vi "front_panel_ctl_save.vi"(0 "VI in":refnum<vi>, 1 "method":enum16{"read controls", "write controls"}(ring), 2 "filename":path, 3 "controls":string[](array[string]), 5 "error in (no error)":errorcluster) -> (8 "error out":errorcluster)   [LabVIEW 2015]
uses:
  <vilib>/Utility/config.llb/Read Key (String).vi
  <vilib>/Utility/config.llb/Write Key (String).vi
  <vilib>/Utility/config.llb/NI_LVConfig.lvlib
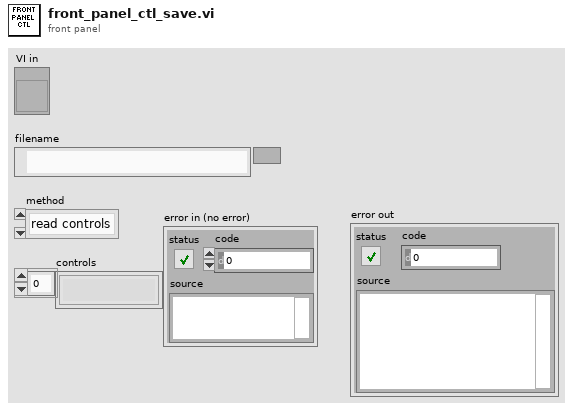
[diagram p1: front panel]
types:
  T1 = typedef "NI_LVConfig.lvlib/Config Data RefNum.ctl" = refnum<k1>
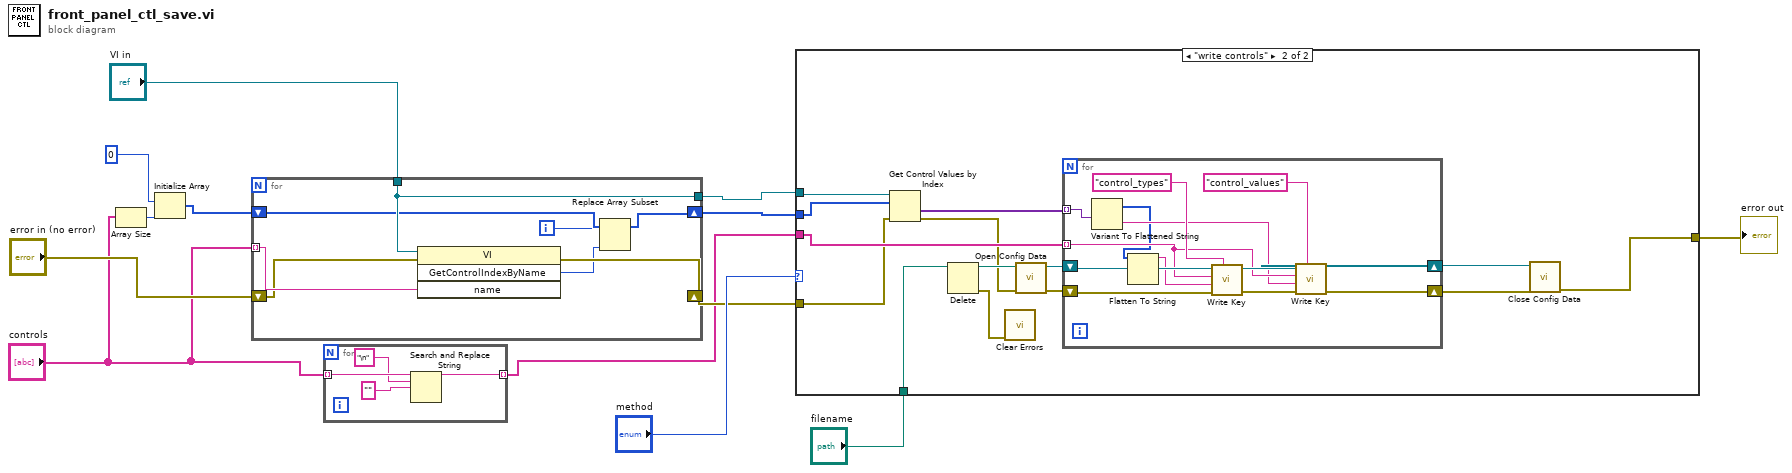
[diagram p0: block diagram]
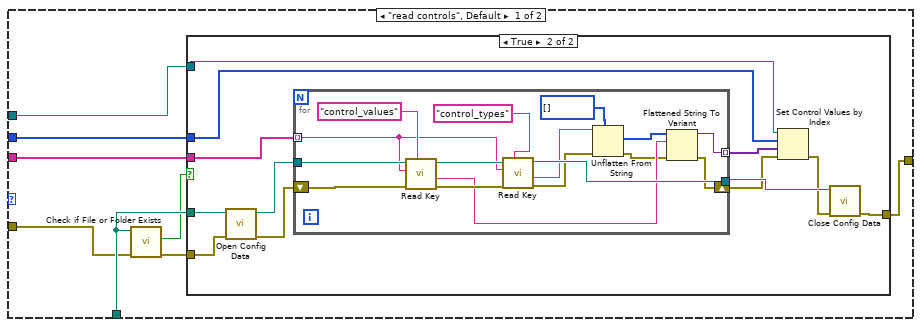
[diagram p2: hidden frame]
diagram:
  n1 = Array Size(array="controls") -> (size(s)=w4:i32)
  n2 = Initialize Array(0 ("Get Control Index by Name"), w4) -> (w2:i32[])
  n3 = for {
    tunnel: "controls" -> [w21] mode=indexing
    shift-right: [w16] -> w12
    shift-left: w2 -> [w17]
    tunnel: [w20] -> w11
    tunnel: "VI in" -> [w20]
    shift-right: [w19] -> w8
    shift-left: "error in (no error)" -> [w18]
    i -> [w15]
    n4 = invoke class="VI" method="GetControlIndexByName"(reference=w20, error in=w18, "name"=w21) -> (error out=w19:errorcluster, "GetControlIndexByName"=w14:i32)  [unwired: 1 in, 2 out]
    n5 = Replace Array Subset(array=w17, new element=w14, index=w15) -> (w16:i32[])
  }
  n6 = for {
    tunnel: "controls" -> [w25] mode=indexing
    tunnel: [w22] -> w5 mode=indexing
    n7 = Search and Replace String(input string=w25, search string="\n", replace string="" ("replace string (\"\")")) -> (result string=w22:string)  [unwired: 5 in, 3 out]
  }
  n8 = case shown="\"write controls\"" "method" {
    tunnel: "filename" -> [w30 w65]
    tunnel: w11 -> [w33 w71]
    tunnel: w12 -> [w32 w72]
    tunnel: w5 -> [w31 w73]
    tunnel: [w26 w70] -> w6
    tunnel: w8 -> [w27 w69]
    frame "read controls", Default {
      n9 = call <vilib>:"Check if File or Folder Exists.vi"("error in (no error)"=w27, "path"=w30) -> ("error out"=w28:errorcluster, "file or folder exists?"=w29:bool)  [unwired: 7 in, 1 out]
      n10 = case shown="True" w29 {
        tunnel: w33 -> [_ w44]
        tunnel: w32 -> [_ w43]
        tunnel: w31 -> [_ w42]
        tunnel: w30 -> [_ w41]
        tunnel: w28 -> [w34 w40]
        tunnel: [w34 w36] -> w26
        frame False {
        }
        frame True {
          n11 = call <vilib>:"Open Config Data.vi"("error in (no error)"=w40, "configuration file path"=w41) -> ("error out"=w45:errorcluster, "refnum"=w46:T1)  [unwired: 7 in, 1 out]
          n12 = for {
            tunnel: w46 -> [w62]
            tunnel: w42 -> [w57] mode=indexing
            tunnel: [w50] -> w39 mode=indexing
            shift-right: [w47] -> w35
            shift-left: w45 -> [w60]
            tunnel: [w55] -> w38
            n13 = call-poly <vilib>:"Read Key.vi"("section"="control_values", "error in (no error)"=w60, "key"=w57, "refnum"=w62) -> ("error out"=w58:errorcluster, "value"=w51:string, "refnum out"=w59:T1)  [unwired: 4 in, 1 out]
            n14 = call-poly <vilib>:"Read Key.vi"("section"="control_types", "error in (no error)"=w58, "key"=w57, "refnum"=w59) -> ("error out"=w48:errorcluster, "value"=w54:string, "refnum out"=w55:T1)  [unwired: 4 in, 1 out]
            n15 = Unflatten From String(type=i16[] [] ("type string"), binary string=w54, error in (no error)=w48) -> (value=w52:i16[], error out=w49:errorcluster)  [unwired: 2 in, 1 out]
            n16 = Flattened String To Variant(4:w49, 6:w51, 7:w52) -> (0:w47:errorcluster, 3:w50:variant)
          }
          n17 = Set Control Values by Index(0:w44, 1:w43, 2:w39, 3:w35) -> (11:w37:errorcluster)
          n18 = call <vilib>:"Close Config Data.vi"("error in (no error)"=w37, "refnum"=w38) -> ("error out"=w36:errorcluster)  [unwired: 8 in, 1 out]
        }
      }
    }
    frame "write controls" {
      n19 = Get Control Values by Index(0:w71, 1:w72, 3:w69) -> (10:w68:variant[], 11:w64:errorcluster)
      n20 = Delete(path (use dialog)=w65) -> (deleted path=w66:path, error out=w63:errorcluster)  [unwired: 4 in, 1 out]
      n21 = call <vilib>:"Clear Errors.vi"("error in (no error)"=w63) -> ()  [unwired: 5 in, 2 out]
      n22 = call <vilib>:"Open Config Data.vi"("error in (no error)"=w64, "configuration file path"=w66) -> ("error out"=w67:errorcluster, "refnum"=w75:T1)  [unwired: 7 in, 1 out]
      n23 = for {
        tunnel: w68 -> [w80] mode=indexing
        tunnel: w73 -> [w81] mode=indexing
        shift-right: [w88] -> w76
        shift-left: w75 -> [w85]
        shift-right: [w89] -> w74
        shift-left: w67 -> [w84]
        n24 = Variant To Flattened String(Variant=w80) -> (data string=w79:string, 1:w77:i16[])
        n25 = Flatten To String(anything=w77) -> (data string=w78:string)  [unwired: 3 in, 2 out]
        n26 = call-poly <vilib>:"Write Key.vi"("section"="control_types", "error in (no error)"=w84, "value"=w78, "key"=w81, "refnum"=w85) -> ("error out"=w86:errorcluster, "refnum out"=w87:T1)  [unwired: 4 in, 1 out]
        n27 = call-poly <vilib>:"Write Key.vi"("section"="control_values", "error in (no error)"=w86, "value"=w79, "key"=w81, "refnum"=w87) -> ("error out"=w89:errorcluster, "refnum out"=w88:T1)  [unwired: 4 in, 1 out]
      }
      n28 = call <vilib>:"Close Config Data.vi"("error in (no error)"=w74, "refnum"=w76) -> ("error out"=w70:errorcluster)  [unwired: 8 in, 1 out]
    }
  }
  "error out" <- w6
